vi "Build Test Result.vi"(8 "error in (no error)":errorcluster, 10 "Report.lvclass":refnum<class "Report.lvclass">, 11 "Test Result in":refnum<class "Test Result.lvclass">) -> (0 "error out":errorcluster)   [LabVIEW 2021, in "Sequence Engine.lvlib" / "Test Step.lvclass"]
uses:
  Test Step.lvclass
  Test Step.lvclass/Test Step.ctl
  Test Result/Test Result.lvclass
  PPLs/Report.lvlibp/Classes/Report/Report.lvclass
  PPLs/Report.lvlibp/Classes/Report/Test Param.ctl
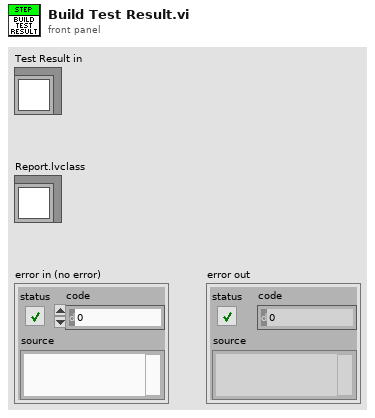
[diagram p1: front panel]
types:
  T1 = typedef "Report.lvlibp/Report.lvclass/Test Param.ctl" = cluster{"Report ID":i32, "Param Name":string, "Expected Value":string, "Value":string, "Test Result":string, "Cycle Time (ms)":dbl}
  T2 = typedef "Sequence Engine.lvlib/Test Result.lvclass/Result Data.ctl" = cluster{"Test ID":u32, "Test Name":string, "Sub Test Name":string, "Test Status":T3, "Start Time":timestamp, "End Time":timestamp, "Duration (s)":dbl, "Expected Values":string, "Measured Values":string, "Remarks":string}
  T3 = typedef "Sequence Engine.lvlib/Test Result.lvclass/Test Status.ctl" = enum16{"Pass", "Fail", "Aborted", "Skipped"}
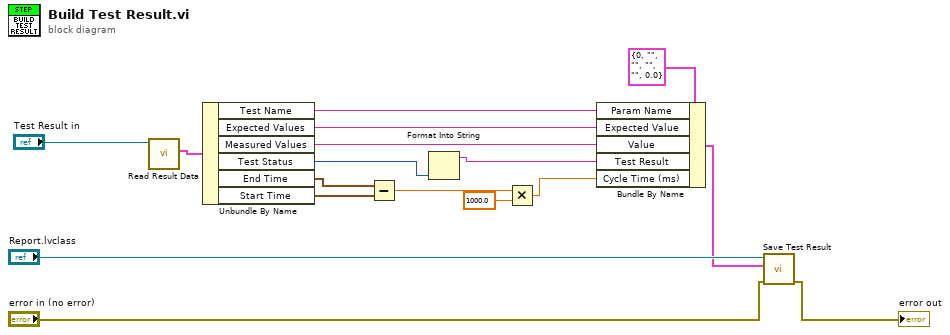
[diagram p0: block diagram]
diagram:
  n1 = call "Read Result Data.vi"("Test Result in"="Test Result in") -> ("Result Data"=w1:T2)  [unwired: 8 in, 2 out]
  n2 = Unbundle By Name(w1) -> ("Test Name"=w2:string, "Expected Values"=w11:string, "Measured Values"=w3:string, "Test Status"=w12:T3, "End Time"=w4:timestamp, "Start Time"=w5:timestamp)
  n3 = Subtract(x=w4, y=w5) -> (x-y=w6:dbl)
  n4 = Format Into String(w12) -> (resulting string=w13:string)  [unwired: 3 in, 1 out]
  n5 = Multiply(x=w6, y=1000.0) -> (x*y=w7:dbl)
  n6 = Bundle By Name(cluster=T1 {"Report ID"=0, "Param Name"="", "Expected Value"="", "Value"="", "Test Result"="", "Cycle Time (ms)"=0.0}, "Param Name"=w2, "Expected Value"=w11, "Value"=w3, "Test Result"=w13, "Cycle Time (ms)"=w7) -> (w10:T1)
  n7 = call "Save Test Result.vi"("error in (no error)"="error in (no error)", "Test Param"=w10, "Report in"="Report.lvclass") -> ("error out"=→"error out":errorcluster)  [unwired: 7 in, 1 out]
